vi "cursor window - init all.vi"(0 "cursor bracket:  Time 2":refnum<vi>, 1 "cursor bracket: fragment 2":refnum<vi>, 2 "cursor bracket:  All, zoom 2":refnum<vi>, 3 "cursor bracket:  All, data window 2":refnum<vi>, 4 "Plot: Time":refnum<vi>, 5 "Plot:  Fragment":refnum<vi>, 6 "cursor bracket:  All, show 2":refnum<vi>, 7 "Plot: All":refnum<vi>) -> ()   [LabVIEW 2015]
uses:
  cursor winow.ctl
  cursor window action.ctl
panel:
  in  "cursor bracket in":T1={"left"=2044.0881763527054, "right "=2126.7657992565055, "center"=2085.4269878046052, "window"=82.67762290380006, "cursors"=[], "relative"=0, "absolute"=0, "fixed vertical offset"=2421.6740576496672, "vertical offset"=2421.6740576496672, "skew"=2421.6740576496672, "default window frac"=2421.6740576496672, "kind"=enum."fancy", "skew.left"=2.0, "skew.right"=0.0, "Plot ref"=refnum, "wing order"=enum."back"}
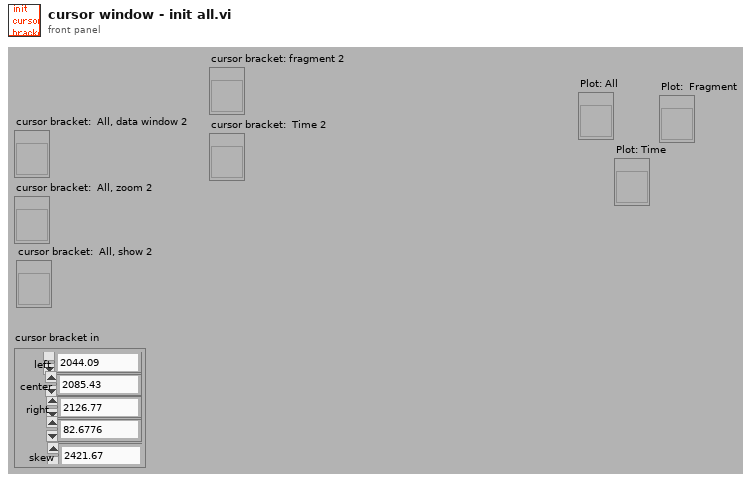
[diagram p1: front panel]
types:
  T1 = typedef "cursor winow.ctl" = cluster{"left":dbl, "right ":dbl, "center":dbl, "window":dbl, "cursors":i32[], "relative":i32, "absolute":i32, "fixed vertical offset":dbl, "vertical offset":dbl, "skew":dbl, "default window frac":dbl, "kind":enum16{"symmetric", "skewed", "fancy"}, "skew.left":dbl, "skew.right":dbl, "Plot ref":refnum<vi>, "wing order":enum16{"forw", "back"}}
  T2 = typedef "cursor window action.ctl" = enum16{"balance", "h. offset change", "cursor moves", "change center", "change window", "init", "check", "reset", "set y to middle", "idle", "-write all Y", "-write left.X", "-write center.X", "-write right.X", "-write all X", "-change center", "-change window", "-change skew", "-read cursor 2", "-read cursor 1", "-read cursor 0", "-read all cursors", "-reset", "-read plot scale", "-set y to middle", "-Q: center.Y is visible", "-Q: window is visible", "-parse center.Y", "-right left from center", "-left move", "-right move", "-set center.Y", "-empty", "-set cursors to default", "-check", "-write center.Y", "-copy cursor 1", "-copy cursor 0", "-copy cursor 2", "move right", "move left", "shrink", "broaden", "skew up", "skew down", "-write plot scale", "zoom X", "change cen&win", "zoom to all data"}
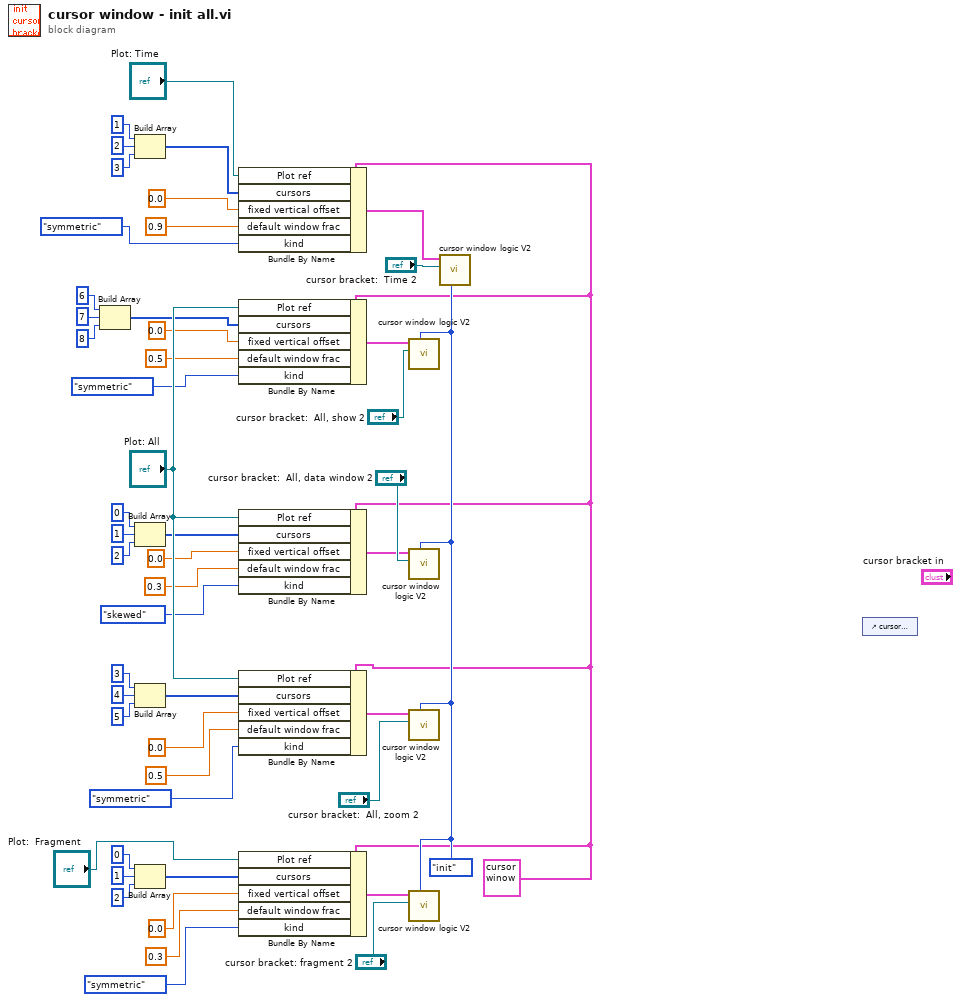
[diagram p0: block diagram]
diagram:
  w1 = T1 {"left"=2044.0881763527054, "right "=2126.7657992565055, "center"=2085.4269878046052, "window"=82.67762290380006, "cursors"=[], "relative"=0, "absolute"=0, "fixed vertical offset"=2421.6740576496672, "vertical offset"=2421.6740576496672, "skew"=2421.6740576496672, "default window frac"=2421.6740576496672, "kind"=enum."fancy", "skew.left"=2.0, "skew.right"=0.0, "Plot ref"=refnum, "wing order"=enum."back"} ("cursor bracket in")
  w2 = cursor_window_action."init" ("cursor window action")
  n1 = Build Array(6, 7, 8) -> (w9:i32[])
  n2 = Build Array(1, 2, 3) -> (w27:i32[])
  n3 = Build Array(0, 1, 2) -> (w41:i32[])
  n4 = Build Array(3, 4, 5) -> (w37:i32[])
  n5 = Build Array(0, 1, 2) -> (w36:i32[])
  n6 = Bundle By Name(cluster=w1, "Plot ref"="Plot: Time", "cursors"=w27, "fixed vertical offset"=0.0, "default window frac"=0.9 ("fixed vertical offset"), "kind"=enum16{"symmetric", "skewed", "fancy"}."symmetric") -> (w26:T1)
  n7 = Bundle By Name(cluster=w1, "Plot ref"="Plot: All", "cursors"=w9, "fixed vertical offset"=0.0, "default window frac"=0.5 ("fixed vertical offset"), "kind"=enum16{"symmetric", "skewed", "fancy"}."symmetric") -> (w10:T1)
  n8 = Bundle By Name(cluster=w1, "Plot ref"="Plot: All", "cursors"=w41, "fixed vertical offset"=0.0, "default window frac"=0.3 ("fixed vertical offset"), "kind"=enum16{"symmetric", "skewed", "fancy"}."skewed") -> (w34:T1)
  n9 = Bundle By Name(cluster=w1, "Plot ref"="Plot: All", "cursors"=w37, "fixed vertical offset"=0.0, "default window frac"=0.5 ("fixed vertical offset"), "kind"=enum16{"symmetric", "skewed", "fancy"}."symmetric") -> (w38:T1)
  n10 = Bundle By Name(cluster=w1, "Plot ref"="Plot:  Fragment", "cursors"=w36, "fixed vertical offset"=0.0, "default window frac"=0.3 ("fixed vertical offset"), "kind"=enum16{"symmetric", "skewed", "fancy"}."symmetric") -> (w35:T1)
  n11 = call "cursor window logic V2.vi"("cursor window action"=w2, "cursor window in"="cursor bracket:  All, show 2", "cursor window init"=w10) -> ()  [unwired: 7 in, 2 out]
  n12 = call "cursor window logic V2.vi"("cursor window action"=w2, "cursor window in"="cursor bracket:  All, data window 2", "cursor window init"=w34) -> ()  [unwired: 7 in, 2 out]
  n13 = call "cursor window logic V2.vi"("cursor window action"=w2, "cursor window in"="cursor bracket:  All, zoom 2", "cursor window init"=w38) -> ()  [unwired: 7 in, 2 out]
  n14 = call "cursor window logic V2.vi"("cursor window action"=w2, "cursor window in"="cursor bracket: fragment 2", "cursor window init"=w35) -> ()  [unwired: 7 in, 2 out]
  n15 = call "cursor window logic V2.vi"("cursor window action"=w2, "cursor window in"="cursor bracket:  Time 2", "cursor window init"=w26) -> ()  [unwired: 7 in, 2 out]
  n16 = control-ref of="cursor bracket in"() -> ()  [unwired: 1 out]
